vi "ConfigureAnalogInputs.vi"(0 "axis in":cluster{"keyHandle":u32, "nodeId":u16}={"keyHandle"=0, "nodeId"=1}, 9 "analog input configuration":T1={"analogInputNumber"=1, "configuration"=15, "executionMask"=0} {"executionMask" items=["Disabled", "Enabled"]; "configuration" items=["current setpoint"=0, "velocity setpoint"=1, "position setpoint"=2, "general purpose A"=15, "general purpose B"=14, "general purpose C"=13, "general purpose D"=12, "general purpose E"=11]}, 11 "error in (no error)":errorcluster) -> (4 "axis out":cluster{"keyHandle":u32, "nodeId":u16}={"keyHandle"=0, "nodeId"=1}, 15 "error out":errorcluster)   [LabVIEW 2018]
doc: "<B>ConfigureAnalogInputs</B> writes the configuration parameters for an analog input to the device."
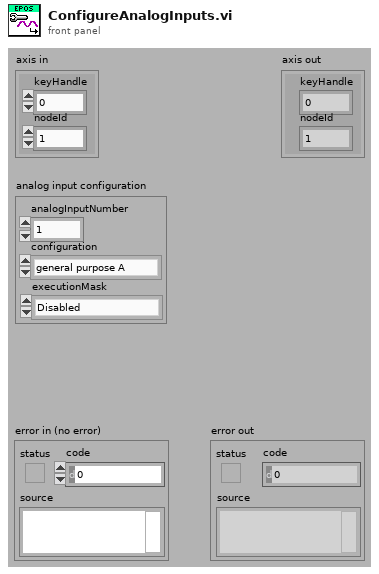
[diagram p1: front panel]
types:
  T1 = cluster{"analogInputNumber":u16, "configuration":u16, "executionMask":i32}
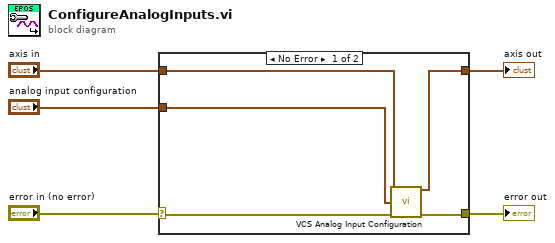
[diagram p0: block diagram]
diagram:
  n1 = case shown="No Error" "error in (no error)" {
    selector: "error in (no error)" -> [w7 w12]
    tunnel: [w10 w12] -> w4
    tunnel: [w9 w11] -> w3
    tunnel: "axis in" -> [w6 w11]
    tunnel: "analog input configuration" -> [w8 _]
    frame No Error {
      n2 = call "VCS Analog Input Configuration.vi"("axis in"=w6, "configuration"=w8, "error in (no error)"=w7) -> ("axis out"=w9:cluster{"keyHandle":u32, "nodeId":u16}, "error out"=w10:errorcluster)  [unwired: 11 in]
    }
    frame Error {
    }
  }
  "error out" <- w4
  "axis out" <- w3
